vi "Update FF_Q.vi"(4 "b0":fxp<+/-,32,2>, 5 "Reset":bool=TRUE, 6 "a0":fxp<+/-,32,2>, 8 "input valid":bool=TRUE, 9 "Buffer size":u32, 10 "destination adress":u32, 11 "source adress":u32) -> (0 "output valid":bool)   [LabVIEW 2018]
uses:
  <vilib>/rvi/Memory/Memory_Emulation/nirvimemoryFastEmulation.vi
  <vilib>/rvi/Memory/Memory_Emulation/nirvimemoryEmulation.vi
  <vilib>/rvi/Emulation/niFpgaEmulationIsFPGAContextNoSignature.vi
  <vilib>/rvi/DataTransferAndStorage/Container/Common/niFpgaContainerGetUniqueNameForEmu.vi
  <vilib>/rvi/Emulation/niFpgaProcessEmulError.vi
  <vilib>/rvi/Emulation/niFpgaSctlEmulationGetInTimedLoop.vi
  <vilib>/rvi/errors/nirviReportUnexpectedCaseInternalError (U32).vi
  <vilib>/rvi/DataTransferAndStorage/Container/XNode/niFpgaContainer.xnode
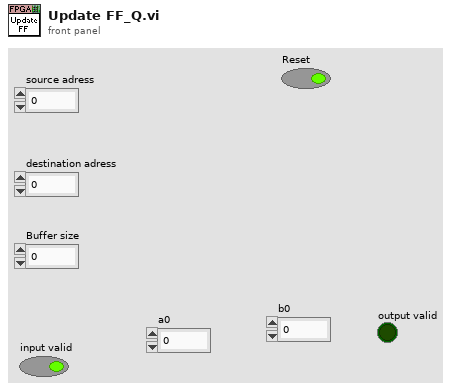
[diagram p1: front panel]
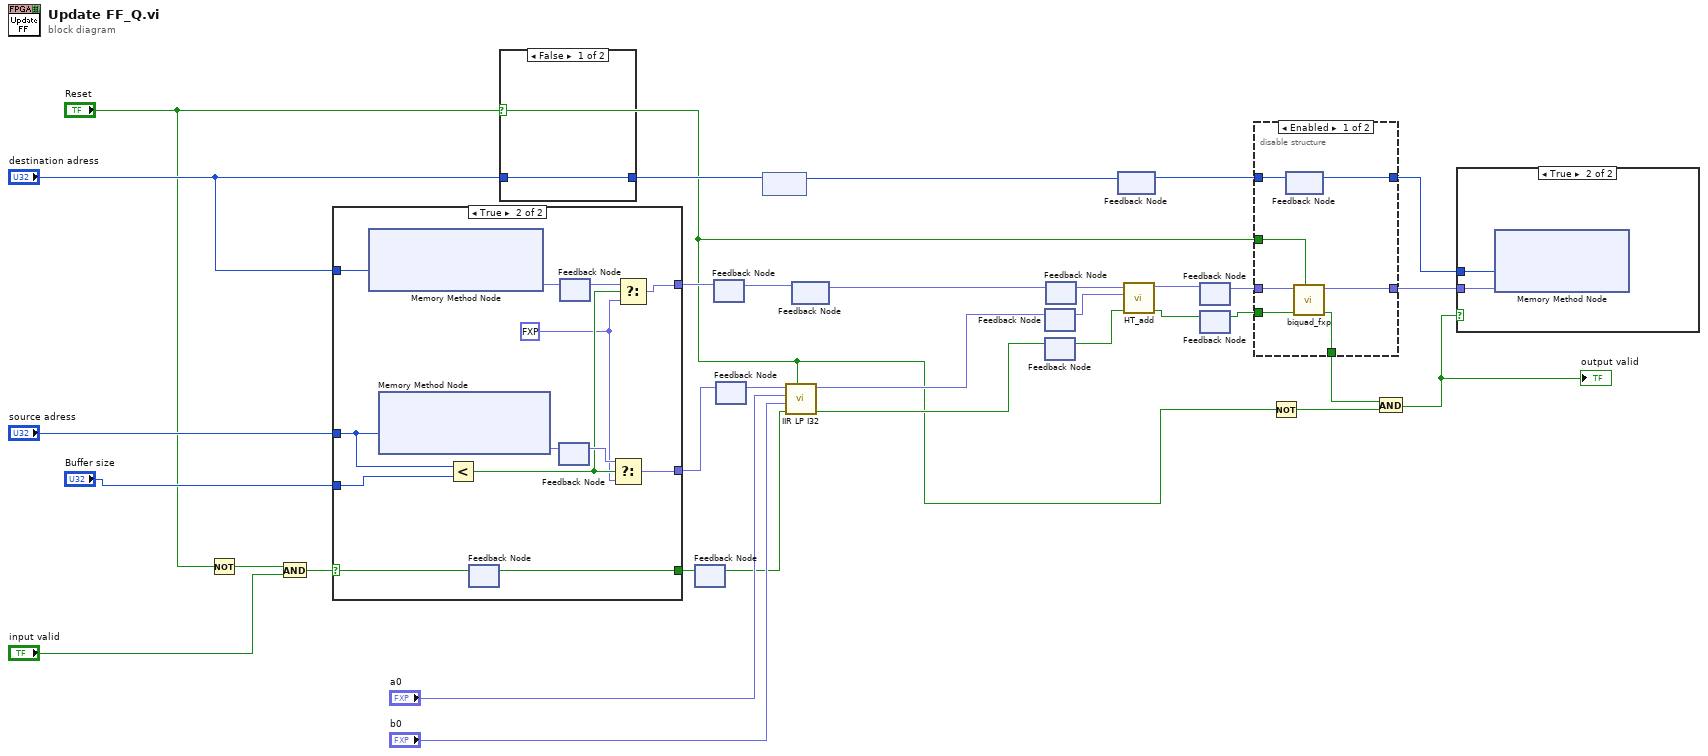
[diagram p0: block diagram]
diagram:
  n1 = Not(x="Reset") -> (.not. x?=w10:bool)
  n2 = And(x=w10, y="input valid") -> (x .and. y?=w8:bool)
  n3 = case shown="True" w8 {
    selector: w8 -> [_ w44]
    tunnel: [_ w38] -> w24
    tunnel: "source adress" -> [_ w42]
    tunnel: [_ w36] -> w22
    tunnel: "destination adress" -> [_ w46]
    tunnel: [_ w43] -> w14
    tunnel: "Buffer size" -> [_ w41]
    frame False {
    }
    frame True {
      w34 = fxp<+/-,32,14> 0.0 ("f")
      n4 = xnode ("Memory Method Node")("Address"=w46) -> ("Data"=w45:fxp<+/-,32,14>)  [unwired: 1 in, 1 out]
      n5 = xnode ("Memory Method Node")("Address"=w42) -> ("Data"=w40:fxp<+/-,32,14>)  [unwired: 1 in, 1 out]
      n6 = Less?(x=w42, y=w41) -> (x < y?=w35:bool)
      n7 = feedback #1() -> (w43:bool)  [unwired: 1 in]
      n8 = feedback-in #1(w44) -> ()
      n9 = feedback #2() -> (w39:fxp<+/-,32,14>)  [unwired: 1 in]
      n10 = feedback-in #2(w40) -> ()
      n11 = feedback #3() -> (w37:fxp<+/-,32,14>)  [unwired: 1 in]
      n12 = feedback-in #3(w45) -> ()
      n13 = Select(t=w39, s=w35, f=w34) -> (s? t:f=w38:fxp<+/-,32,14>)
      n14 = Select(t=w37, s=w35, f=w34) -> (s? t:f=w36:fxp<+/-,32,14>)
    }
  }
  n15 = case shown="False" "Reset" {
    tunnel: "destination adress" -> [w47 _]
    tunnel: [w47 _] -> w16
    frame False {
    }
    frame True {
    }
  }
  n16 = feedback #4() -> (w15:bool)  [unwired: 1 in]
  n17 = feedback-in #4(w14) -> ()
  n18 = feedback #5() -> (w21:fxp<+/-,32,14>)  [unwired: 1 in]
  n19 = feedback-in #5(w22) -> ()
  n20 = feedback-in #6(w24) -> ()
  n21 = feedback #6() -> (w27:fxp<+/-,32,14>)  [unwired: 1 in]
  n22 = feedback #7() -> (w18:u32)  [unwired: 1 in]
  n23 = feedback-in #7(w16) -> ()
  n24 = call "IIR LP I32.vi"("Reset"="Reset", "input valid"=w15, "b0"="b0", "a0"="a0", "Value in"=w27) -> ("output valid"=w23:bool, "Value out"=w26:fxp<+/-,32,14>)  [unwired: 5 in]
  n25 = feedback #8() -> (w20:fxp<+/-,32,14>)  [unwired: 1 in]
  n26 = feedback-in #8(w21) -> ()
  n27 = feedback #9() -> (w28:fxp<+/-,32,14>)  [unwired: 1 in]
  n28 = feedback-in #9(w26) -> ()
  n29 = feedback #10() -> (w31:bool)  [unwired: 1 in]
  n30 = feedback-in #10(w23) -> ()
  n31 = feedback #11() -> (w19:fxp<+/-,32,14>)  [unwired: 1 in]
  n32 = feedback-in #11(w20) -> ()
  n33 = feedback #12() -> (w3:u32)  [unwired: 1 in]
  n34 = feedback-in #12(w18) -> ()
  n35 = call "HT_add.vi"("input valid"=w31, "y"=w28, "x"=w19) -> ("output valid"=w29:bool, "x+y"=w30:fxp<+/-,32,14>)  [unwired: 7 in]
  n36 = feedback #13() -> (w6:fxp<+/-,32,14>)  [unwired: 1 in]
  n37 = feedback-in #13(w30) -> ()
  n38 = feedback #14() -> (w4:bool)  [unwired: 1 in]
  n39 = feedback-in #14(w29) -> ()
  n40 = disable-structure shown="Enabled" {
    disable-tunnel: [w54 w55] -> w7
    disable-tunnel: w6 -> [w53 w56]
    disable-tunnel: [w52 w56] -> w5
    disable-tunnel: w4 -> [w51 w55]
    disable-tunnel: w3 -> [w50 w57]
    disable-tunnel: [w49 w57] -> w2
    disable-tunnel: "Reset" -> [w48 _]
    frame Enabled {
      n41 = feedback #15() -> (w49:u32)  [unwired: 1 in]
      n42 = feedback-in #15(w50) -> ()
      n43 = call "biquad_fxp.vi"("reset"=w48, "input valid"=w51, "x"=w53) -> ("output valid"=w54:bool, "y"=w52:fxp<+/-,32,14>)  [unwired: 7 in]
    }
    frame Disabled {
    }
  }
  n44 = Not(x="Reset") -> (.not. x?=w25:bool)
  n45 = And(x=w7, y=w25) -> (x .and. y?=w13:bool)
  "output valid" <- w13
  n46 = case shown="True" w13 {
    tunnel: w5 -> [_ w59]
    tunnel: w2 -> [_ w58]
    frame False {
    }
    frame True {
      n47 = xnode ("Memory Method Node")("Address"=w58, "Data"=w59) -> ()  [unwired: 1 in, 1 out]
    }
  }
